vi "Write CD Template.vi"(8 "error in (no error)":errorcluster, 10 "CD Template":refnum<class "NIVS_CD Template.lvclass">, 11 "NIVS_Consolidated_CDW_MetaDataObj in":refnum<class "NIVS_Consolidated_CDW_MetaDataObj.lvclass">) -> (0 "error out":errorcluster, 3 "NIVS_Consolidated_CDW_MetaDataObj out":refnum<class "NIVS_Consolidated_CDW_MetaDataObj.lvclass">)   [LabVIEW 2015, in "NIVS_Consolidated_CDW_MetaDataObj.lvclass"]
uses:
  NIVS_Consolidated_CDW_MetaDataObj.lvclass
  Template Classes/NIVS_CD Template/NIVS_CD Template.lvclass
  NIVS_Consolidated_CDW_MetaDataObj.lvclass/NIVS_Consolidated_CDW_MetaDataObj.ctl
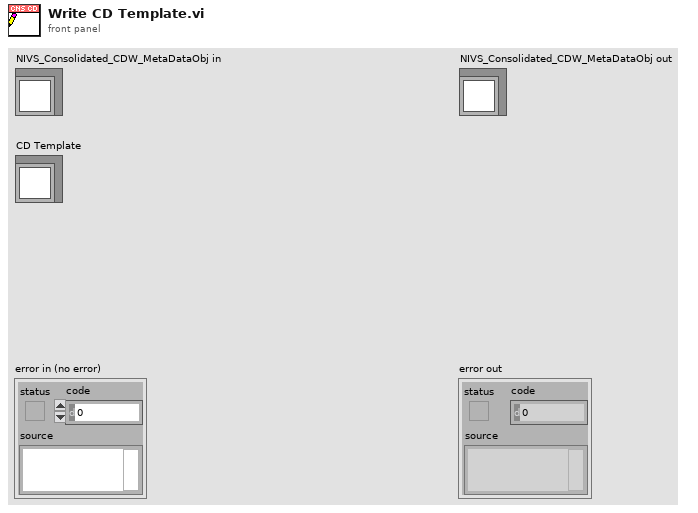
[diagram p1: front panel]
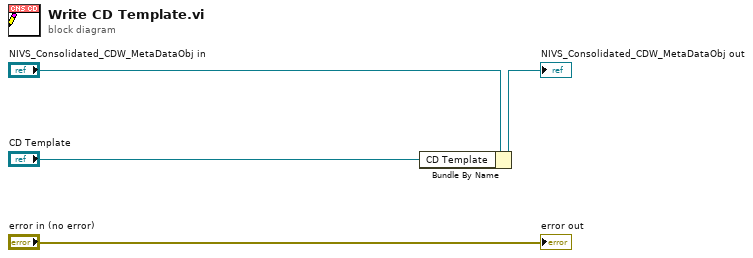
[diagram p0: block diagram]
diagram:
  n1 = Bundle By Name(cluster="NIVS_Consolidated_CDW_MetaDataObj in", "CD Template"="CD Template") -> (→"NIVS_Consolidated_CDW_MetaDataObj out":refnum<class "NIVS_Consolidated_CDW_MetaDataObj.lvclass">)
  "error out" <- "error in (no error)"
